vi "RVC Drive Cartesian Maneuver.vi"() -> ()   [LabVIEW 2017]
uses:
  <vilib>/Simulation/Scripting/Companion Diagram/SimConfigNode/SimParams.ctl
  <vilib>/Simulation/Scripting/Companion Diagram/SimConfigNode/_simSolvers.ctl
  <vilib>/Simulation/Implementation/Shared/SIMSCR Execution Mode.ctl
  <vilib>/Simulation/Param Hierarchy/Typedefs/SIMPH Param Control Actions.ctl
  <vilib>/Simulation/Scripting/Editor Utilities/SIM subVI tag data.ctl
  <vilib>/Simulation/Scripting/Editor Utilities/SIM subVI execution type.ctl
  <vilib>/Simulation/Implementation/Shared/NILVSim_ParamChanged.vi
  <vilib>/Simulation/Implementation/Shared/NILVSIM_BeginStep.vi
  <vilib>/Simulation/Utility/Implementation/SIM Time.vi
  <vilib>/Simulation/SignalArithmetic/Implementation/NILVSim Gain.llb/SIM Gain (scalar).vi
  <vilib>/Simulation/Utility/Implementation/NILVSim Collector.llb/SIM Collector (vector).vi
  <vilib>/Simulation/Utility/Implementation/NILVSim Collector.llb/SIM Collector (scalar).vi
  <vilib>/Analysis/coordinate.llb/Wrap Angle.vi
  <vilib>/Analysis/coordinate.llb/Wrap Angle (scalar).vi
  <vilib>/Simulation/Implementation/Shared/SIM Fire Discrete SubVI.vi
  <vilib>/Simulation/Implementation/Shared/NILVSim_Manager.vi
  <vilib>/Utility/error.llb/Clear Errors.vi
  <vilib>/Simulation/Implementation/Shared/NILVSim_FinalizeModel.vi
  <vilib>/Simulation/Utility/Implementation/NILVSim Collector.llb/NILVSim Collector core (vector).vi
  <vilib>/Simulation/Utility/Implementation/NILVSim Collector.llb/NILVSim Collector core (scalar).vi
  <vilib>/Simulation/Implementation/Shared/SIM Fire Discrete SubVI (Core).vi
  <vilib>/Simulation/Implementation/Shared/SIM Unbundle Sim Info.vi
  <vilib>/Simulation/Implementation/Shared/NILVSim_Initialize.vi
  <vilib>/Simulation/Utility/Implementation/NILVSim Get Time and IsAcceptedStep.vi
  <vilib>/addons/control/pid/pid.llb/PID Output Rate Limiter.vi
  <vilib>/addons/control/pid/pid.llb/PID Output Rate Limiter (DBL).vi
  penguin/lvaddon/robotics/branches/untargeted/Bordeaux/Book/Chapter 4/subVIs/2D Animate Rotating Wheel.vi
  penguin/lvaddon/robotics/branches/untargeted/Bordeaux/Book/Chapter 4/subVIs/2D Animation Plot.vi
  <vilib>/Simulation/Implementation/Shared/SIMSH Read Queue.vi
  <vilib>/Simulation/Implementation/Shared/NILVSim_GetModelError.vi
  <vilib>/Simulation/Implementation/Shared/SIM Bundle Sim Info.vi
  <vilib>/Simulation/Scripting/Companion Diagram/SimConfigNode/SimDog.xnode
  penguin/lvaddon/robotics/branches/untargeted/Bordeaux/Book/Chapter 4/SIM Bicycle.vi
  <vilib>/Simulation/Model Libraries/PID/SIM PID (Parallel).vi
  <vilib>/Simulation/Model Libraries/PID/SIM PID.vi
  <vilib>/Simulation/Implementation/XNodeFramework/SimXNode/SimX.xnode
  <vilib>/Analysis/NI_AAL_Angle.lvlib
  <vilib>/addons/control/pid/NI_PID_pid.lvlib
  <vilib>/Simulation/Implementation/Shared/NI_SIM_Implementation.lvlib
panel:
  in  "output rate limit":dbl=55.0 format="%#_13g"
  out "Angle":cluster{"Time":dbl[], "Signal":dbl[]}(graph)
  in  "target radius":dbl=2.0 format="%#_13g"
  in  "target speed":dbl=0.1 format="%#_13g"
  out "Coordinate Frame":cluster{dbl[], dbl[]}[](graph)
  out "Speed":cluster{"Time":dbl[], "Signal":dbl[]}(graph)
  out "Position":cluster{"Signal":dbl[], "Signal":dbl[]}(graph)
  out "Position":cluster{"x":dbl, "y":dbl, "theta":dbl}
  out "Angle (deg)":dbl format="%.2f"
  out "Steering Angle":picture
  out "Goal":dbl[](array[numeric])
  out "velocity":dbl(knob)=1.0 scale=0.0..10.0
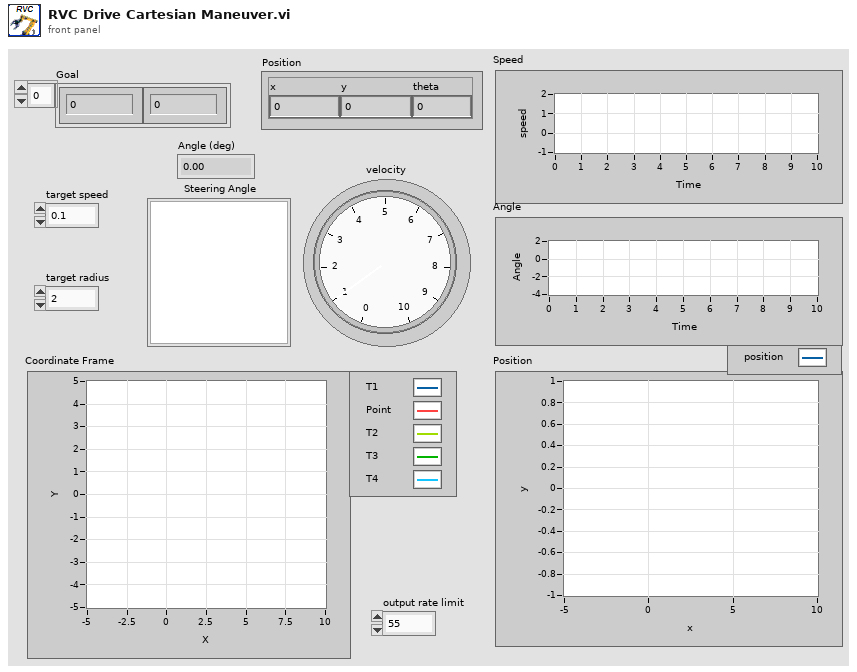
[diagram p1: front panel]
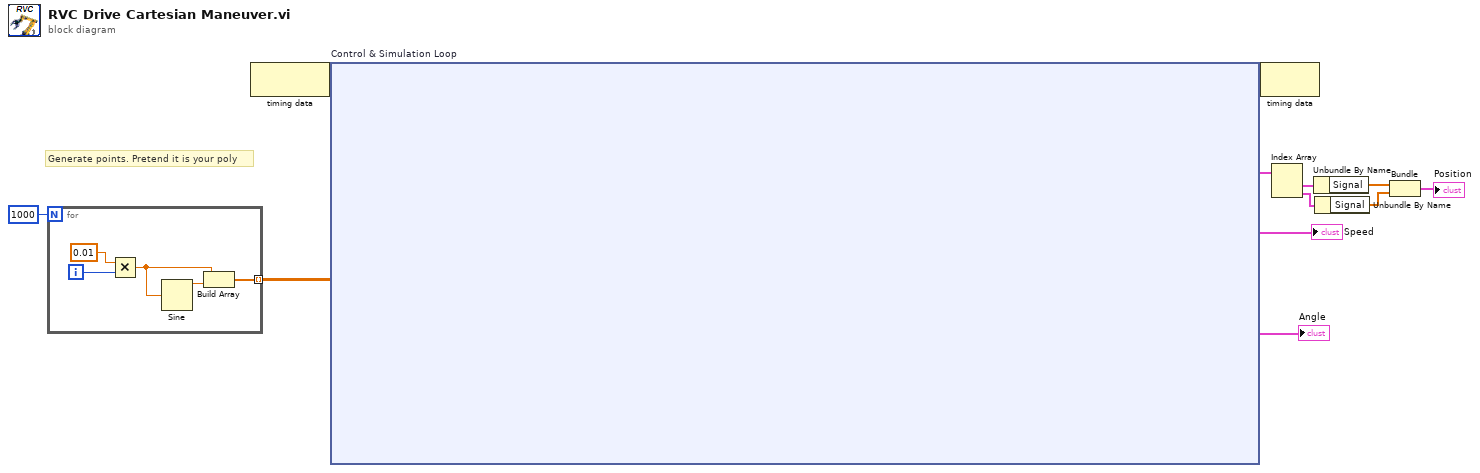
[diagram p0: block diagram]
diagram:
  # "Generate points. Pretend it is your poly"
  n1 = for {
    N: 1000 -> [_]
    tunnel: [w13] -> w2 mode=indexing
    i -> [w17]
    n2 = Multiply(x=0.01 ("y"), y=w17) -> (x*y=w15:dbl)
    n3 = Sine(x=w15) -> (sin(x)=w14:dbl)
    n4 = Build Array(w15, w14) -> (w13:dbl[])
  }
  n5 = node-c288() -> (w11:variant)  [unwired: 1 in]
  n6 = node-c254 "Control & Simulation Loop"(w11, w2) -> (w10:variant, w9:cluster{"Time":dbl[], "Signal":dbl[]}[], →"Speed":cluster{"Time":dbl[], "Signal":dbl[]}, →"Angle":cluster{"Time":dbl[], "Signal":dbl[]})
  n7 = node-c288(w10) -> ()  [unwired: 1 out]
  n8 = Index Array(array=w9) -> (element #1=w8:cluster{"Time":dbl[], "Signal":dbl[]}, element #2=w7:cluster{"Time":dbl[], "Signal":dbl[]})  [unwired: 2 in]
  n9 = Unbundle By Name(w8) -> ("Signal"=w6:dbl[])
  n10 = Unbundle By Name(w7) -> ("Signal"=w5:dbl[])
  n11 = Bundle("Signal"=w6, "Signal"=w5) -> (→"Position":cluster{"Signal":dbl[], "Signal":dbl[]})  [unwired: 1 in]
